vi "SVL AC & DC Level (1 Ch DBL Array).vi"(9 "window":u16(ring)=8 items=["None ", "Hanning", "Hamming", "Blackman-Harris", "Exact Blackman", "Blackman", "Flat Top", "4 Term B-Harris ", "7 Term B-Harris", "Low Sidelobe"], 11 "scaled signal [EU]":dbl[](array[numeric])) -> (1 "DC level [EU]":dbl=nan format="%0.2f", 2 "AC level [EU rms]":dbl=nan format="%.8f", 3 "AC signal [EU]":dbl[](array[numeric]))   [LabVIEW 2017]
doc: "Computes the AC level and DC level of a signal. Wire data to the <B>scaled signal [EU]</B> input to determine the polymorphic instance to use or manually select the instance."
uses:
  <vilib>/Analysis/baseanly.llb/Mean (DBL).vi
  <vilib>/Analysis/0measdsp.llb/Scaled Time Domain Window (DBL).vi
  <vilib>/Analysis/NI_AALBase.lvlib
  <vilib>/Analysis/NI_AALPro.lvlib
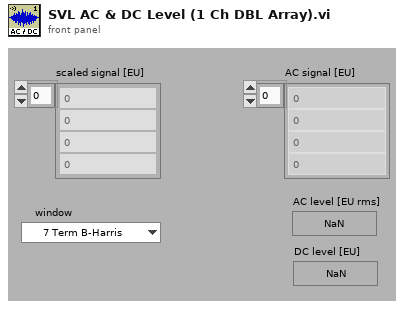
[diagram p1: front panel]
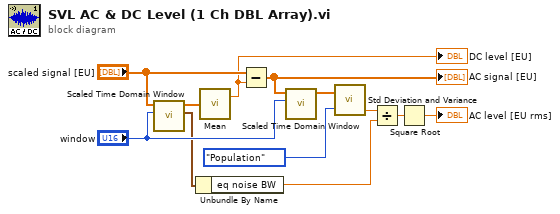
[diagram p0: block diagram]
diagram:
  n1 = call-poly <vilib>:"Scaled Time Domain Window.vi"("window"="window", "X"="scaled signal [EU]") -> ("window properties"=w8:cluster{"eq noise BW":dbl, "coherent gain":dbl}, "Windowed X"=w3:dbl[])  [unwired: 7 in, 1 out]
  n2 = Unbundle By Name(w8) -> ("eq noise BW"=w4:dbl)
  n3 = call-poly <vilib>:"Mean.vi"("X"=w3) -> ("mean"=w9:dbl)  [unwired: 1 out]
  "DC level [EU]" <- w9
  n4 = Subtract(x="scaled signal [EU]", y=w9) -> (x-y=w1:dbl[])
  "AC signal [EU]" <- w1
  n5 = call-poly <vilib>:"Scaled Time Domain Window.vi"("window"="window", "X"=w1) -> ("Windowed X"=w2:dbl[])  [unwired: 7 in, 2 out]
  n6 = call <vilib>:"Std Deviation and Variance.vi"("X"=w2, "Weighting (Sample)"=enum16{"Sample", "Population"}."Population") -> ("variance"=w7:dbl)  [unwired: 2 out]
  n7 = Divide(x=w7, y=w4) -> (x/y=w5:dbl)
  n8 = Square Root(x=w5) -> (sqrt(x)=→"AC level [EU rms]":dbl)
